vi "PCO_RecorderResetLib.vi"(8 "error in (no error)":errorcluster {"code" format="%x"}, 10 "bSilent":bool) -> (0 "error out":errorcluster {"code" format="%x"}, 2 "ErrorMessage":i32 format="%x")   [LabVIEW 2019, in "Recorder.lvlib"]
doc: "<b>Description:</b>\nThis function checks if a recorder instance is active. If so, the user is asked whether he really wants to reset. If the silent flag is set, this Message Box will be omitted and reset will be done either way.\n\n<b>Supported camera type:</b>\nAll cameras"
uses:
  Recorder.lvlib
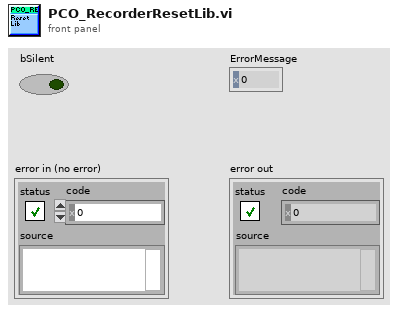
[diagram p1: front panel]
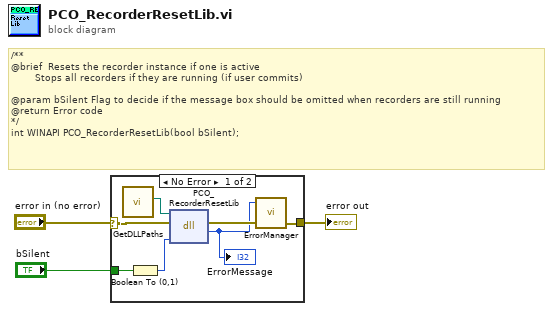
[diagram p0: block diagram]
diagram:
  # "/**\n@brief \tResets the recorder instance if one is active\n        Stops all recorders if they are running (if user commits)\n\n@param bSilent Flag to decide if the message box should be omitted when recorders are still running\n@return Error code\n*/\nint WINAPI PCO_RecorderResetLib(bool bSilent);"
  n1 = case shown="No Error" "error in (no error)" {
    selector: "error in (no error)" -> [w8 w11]
    tunnel: "bSilent" -> [w10 _]
    tunnel: [w7 w11] -> w2
    frame No Error {
      n2 = call "GetDLLPaths.vi"() -> ("PCO_Recorder_Path"=w4:path)  [unwired: 8 in, 3 out]
      n3 = Boolean To (0,1)(Boolean=w10) -> (0, 1=w9:i16)
      n4 = dll-call lib="?" fn="PCO_RecorderResetLib"(path in=w4, error in=w8, "bSilent"=w9) -> (error out=w6:errorcluster, "return type"=w5:i32)  [unwired: 2 in, 1 out]
      "ErrorMessage" <- w5
      n5 = call "ErrorManager.vi"("error in (no error)"=w6, "error code"=w5) -> ("error out"=w7:errorcluster)  [unwired: 2 in, 1 out]
    }
    frame Error {
    }
  }
  "error out" <- w2
